vi "Read.vi"(8 "error in (no error)":errorcluster, 10 "Name":string, 11 "TwinCAT ADS in":refnum<class "TwinCAT ADS.lvclass">) -> (0 "error out":errorcluster, 1 "Value":variant, 3 "TwinCAT ADS out":refnum<class "TwinCAT ADS.lvclass">)   [LabVIEW 2018, in "TwinCAT ADS.lvclass"]
uses:
  TwinCAT ADS.lvclass
  TwinCAT.Ads
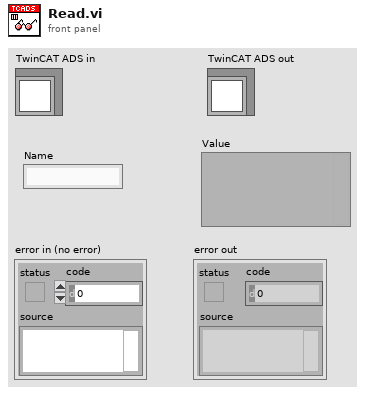
[diagram p1: front panel]
types:
  T1 = typedef "TwinCAT ADS.lvclass/Symbol Information.ctl" = cluster{"Name":string, "Short Name":string, "Size":i32, "Type Category":i32, "Type Name":string, "Type ID":i32, "Index Group":i64, "Index Offset":i64, "Child Count":i32, "Has Rpc Methods?":bool, "Comment":string}
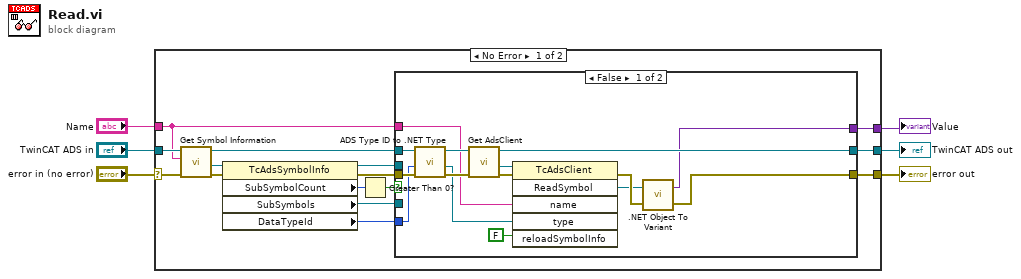
[diagram p0: block diagram]
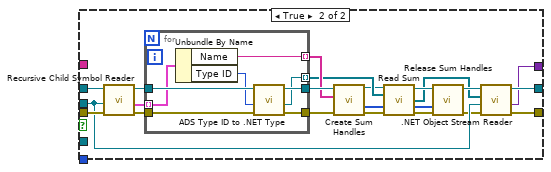
[diagram p2: hidden frame]
diagram:
  n1 = case shown="No Error" "error in (no error)" {
    selector: "error in (no error)" -> [w19 w68]
    tunnel: [w12 w68] -> w5
    tunnel: [w11 w67] -> w3
    tunnel: "TwinCAT ADS in" -> [w8 w67]
    tunnel: "Name" -> [w7 _]
    tunnel: [w10 _] -> w1
    frame No Error {
      n2 = call-dynamic "Get Symbol Information.vi"("error in (no error)"=w19, "Name"=w7, "TwinCAT ADS in"=w8) -> ("error out"=w21:errorcluster, "Symbol Info"=w20:refnum<k24>, "TwinCAT ADS out"=w16:refnum<class "TwinCAT ADS.lvclass">)  [unwired: 6 in]
      n3 = property class="TcAdsSymbolInfo"(reference=w20, error in=w21) -> (reference out=w9:refnum<k24>, error out=w17:errorcluster, "SubSymbolCount"=w13:i32, "SubSymbols"=w14:refnum<k24>, "DataTypeId"=w15:i32)
      n4 = Greater Than 0?(x=w13) -> (x > 0?=w18:bool)
      n5 = case shown="False" w18 {
        tunnel: w17 -> [w35 w49]
        tunnel: w16 -> [w34 w48]
        tunnel: w15 -> [w33 _]
        tunnel: w14 -> [_ _]
        tunnel: w7 -> [w28 _]
        tunnel: [w24 w38] -> w12
        tunnel: [w23 w39] -> w11
        tunnel: [w22 w37] -> w10
        tunnel: w9 -> [_ w41]
        frame False {
          n6 = call "ADS Type ID to .NET Type.vi"("error in (no error)"=w35, "Type ID"=w33, "TwinCAT ADS in"=w34) -> ("error out"=w31:errorcluster, ".NET Type"=w29:refnum<k24>, "TwinCAT ADS out"=w30:refnum<class "TwinCAT ADS.lvclass">)  [unwired: 6 in]
          n7 = call-dynamic "Get AdsClient.vi"("error in (no error)"=w31, "TwinCAT ADS in"=w30) -> ("error out"=w36:errorcluster, ".NET TcAdsClient refnum"=w25:refnum<k24>, "TwinCAT ADS out"=w23:refnum<class "TwinCAT ADS.lvclass">)  [unwired: 7 in]
          n8 = invoke class="TcAdsClient" method="ReadSymbol"(reference=w25, error in=w36, "name"=w28, "type"=w29, "reloadSymbolInfo"=FALSE) -> (error out=w27:errorcluster, "ReadSymbol"=w26:refnum<k24>)  [unwired: 1 in, 4 out]
          n9 = call <vilib>:".NET Object To Variant.vi"("error in (no error)"=w27, ".NET object"=w26) -> ("error out"=w24:errorcluster, "variant"=w22:variant)
        }
        frame True {
          n10 = call "Recursive Child Symbol Reader.vi"("error in (no error)"=w49, ".NET TcAdsSymbolInfo"=w41, "TwinCAT ADS in"=w48) -> ("error out"=w47:errorcluster, "Symbols Information"=w45:T1[], "TwinCAT ADS out"=w46:refnum<class "TwinCAT ADS.lvclass">)  [unwired: 6 in]
          n11 = for {
            tunnel: w45 -> [w64] mode=indexing
            tunnel: w47 -> [w66]
            tunnel: [w62] -> w56 mode=indexing
            tunnel: [w60] -> w58
            tunnel: w46 -> [w65]
            tunnel: [w61] -> w57
            tunnel: [w59] -> w53 mode=indexing
            n12 = Unbundle By Name(w64) -> ("Name"=w62:string, "Type ID"=w63:i32)
            n13 = call "ADS Type ID to .NET Type.vi"("error in (no error)"=w66, "Type ID"=w63, "TwinCAT ADS in"=w65) -> ("error out"=w60:errorcluster, ".NET Type"=w59:refnum<k24>, "TwinCAT ADS out"=w61:refnum<class "TwinCAT ADS.lvclass">)  [unwired: 6 in]
          }
          n14 = call-dynamic "Create Sum Handles.vi"("error in (no error)"=w58, "Names"=w56, "TwinCAT ADS in"=w57) -> ("error out"=w55:errorcluster, "Handles"=w54:u32[], "TwinCAT ADS out"=w44:refnum<class "TwinCAT ADS.lvclass">)  [unwired: 6 in]
          n15 = call-dynamic "Read Sum.vi"("TwinCAT ADS in"=w44, ".NET Type Stream"=w53, "Handles"=w54, "error in (no error)"=w55) -> ("TwinCAT ADS out"=w50:refnum<class "TwinCAT ADS.lvclass">, ".NET Object Stream"=w42:refnum<k24>[], "Handles"=w51:u32[], "error out"=w52:errorcluster)  [unwired: 8 in]
          n16 = call-dynamic "Release Sum Handles.vi"("error in (no error)"=w52, "Handles"=w51, "TwinCAT ADS in"=w50) -> ("error out"=w40:errorcluster, "TwinCAT ADS out"=w43:refnum<class "TwinCAT ADS.lvclass">)  [unwired: 7 in]
          n17 = call-dynamic ".NET Object Stream Reader.vi"("error in (no error)"=w40, ".NET TcAdsSymbolInfo"=w41, ".NET Object Stream"=w42, "TwinCAT ADS in"=w43) -> ("error out"=w38:errorcluster, "G Object"=w37:variant, "TwinCAT ADS out"=w39:refnum<class "TwinCAT ADS.lvclass">)  [unwired: 5 in]
        }
      }
    }
    frame Error {
    }
  }
  "error out" <- w5
  "TwinCAT ADS out" <- w3
  "Value" <- w1
